vi "Control main.vi"(11 "chosen  distance":dbl) -> ()   [LabVIEW 2015]
uses:
  <vilib>/myRIO/Instrument Drivers/Onboard IO/PWM/typedefs/PWM Reference.ctl
  <vilib>/myRIO/Common/Instrument Driver Framework/Utilities/typedefs/myRIO Generic Hardware Reference.ctl
  <vilib>/myRIO/Common/Instrument Driver Framework/Utilities/typedefs/Hardware Version Enum.ctl
  <vilib>/myRIO/Common/Instrument Driver Framework/Utilities/typedefs/myRIO v1.0 Reference.ctl
  <vilib>/myRIO/Common/Instrument Driver Framework/Utilities/typedefs/Generic FPGA Reference.ctl
  <vilib>/myRIO/Common/Instrument Driver Framework/myRIO v1.0/PWM/typedefs/PWM Channels Enum.ctl
  <vilib>/myRIO/Instrument Drivers/Onboard IO/PWM/typedefs/PWM Configuration.ctl
  <vilib>/userdefined/High Color/nirio_resource_hc.ctl
  <vilib>/myRIO/Common/Instrument Driver Framework/Utilities/vis/Is FPGA Ref Available.vi
  <vilib>/myRIO/Common/Instrument Driver Framework/myRIO v1.0/PWM/vis/myRIO v1.1 Open PWM.vi
  <vilib>/myRIO/Instrument Drivers/Onboard IO/PWM/vis/Set Duty Cycle and Frequency.vi
  <vilib>/myRIO/Common/Instrument Driver Framework/Utilities/vis/Validate Channels.vi
  <vilib>/myRIO/Common/Instrument Driver Framework/myRIO v1.0/PWM/vis/myRIO v1.0 Reserve PWM.vi
  <vilib>/myRIO/Common/Instrument Driver Framework/myRIO v1.0/PWM/vis/myRIO v1.0 Build MUX Configuration PWM.vi
  <vilib>/myRIO/Common/Instrument Driver Framework/myRIO v1.0/Resource Manager/vis/myRIO v1.0 Reserve Channel List.vi
  <vilib>/myRIO/Common/Instrument Driver Framework/myRIO v1.0/Resource Manager/vis/myRIO v1.0 Create Configuration List.vi
  <vilib>/myRIO/Common/Instrument Driver Framework/myRIO v1.0/Resource Manager/vis/myRIO v1.0 Reserve Channel.vi
  <vilib>/myRIO/Common/Instrument Driver Framework/myRIO v1.0/Resource Manager/vis/myRIO v1.0 Unreserve Channel.vi
  <vilib>/myRIO/Common/Instrument Driver Framework/myRIO v1.0/Resource Manager/vis/myRIO v1.0 Build Mutex Name.vi
  <vilib>/Utility/VariantDataType/GetNumericInfo.vi
  <vilib>/Utility/error.llb/Error Cluster From Error Code.vi
  <vilib>/myRIO/Common/Instrument Driver Framework/myRIO v1.0/myRIO v1.1 Open.vi
  <vilib>/myRIO/Common/Instrument Driver Framework/Utilities/vis/IO Manager.vi
  <vilib>/myRIO/Common/Instrument Driver Framework/Utilities/vis/Configuration Manager.vi
  <vilib>/myRIO/Common/Instrument Driver Framework/myRIO v1.0/Resource Manager/vis/myRIO v1.0 Configure IO.vi
  <vilib>/myRIO/Common/Instrument Driver Framework/myRIO v1.0/myRIO v1.0 Close.vi
  <vilib>/myRIO/Common/Instrument Driver Framework/myRIO v1.0/PWM/vis/myRIO v1.0 Write PWM.vi
  <vilib>/myRIO/Express VI/Onboard IO/PWM/PWM Express VI.xnode
  <vilib>/myRIO/Instrument Drivers/Onboard IO/PWM/vis/myRIO PWM Open.xnode
  <vilib>/myRIO/Instrument Drivers/Onboard IO/PWM/PWM.lvlib
panel:
  in  "error in (no error) 2":errorcluster
  out "error out 5":errorcluster
  out "error out 4":errorcluster
  out "Current location":dbl
  out "First location":dbl
  out "Final location":dbl
  out "remainder":dbl
  out "error out":errorcluster
  in  "error in (no error)":errorcluster
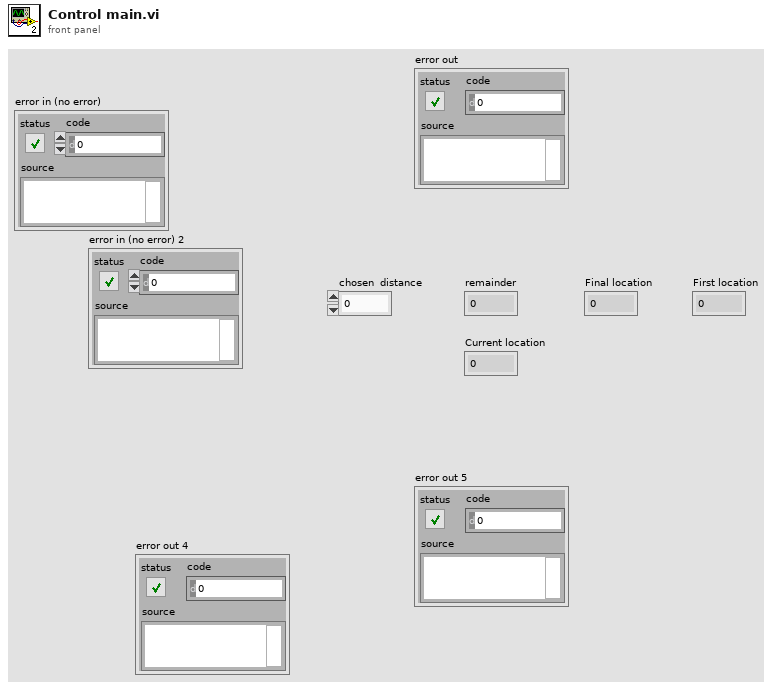
[diagram p1: front panel]
types:
  T1 = typedef "PWM.lvlib/PWM Reference.ctl" = cluster{"myRIO Reference":T2, "PWM Channels Enum":T6, "PWM Configuration":T7}
  T2 = typedef "myRIO Generic Hardware Reference.ctl" = cluster{"myRIO Model":T3, "myRIO Hardware Reference":T4}
  T3 = typedef "Hardware Version Enum.ctl" = enum16{"Unknown", "myRIO-1900", "myRIO-1950", "roboRIO"}
  T4 = typedef "myRIO v1.0 Reference.ctl" = cluster{"Generic FPGA Reference":T5, "Allow multiple opens":bool}
  T5 = typedef "Generic FPGA Reference.ctl" = refnum<k20>
  T6 = typedef "PWM Channels Enum.ctl" = enum16{"Not Connected", "C/PWM0", "C/PWM1", "A/PWM0", "A/PWM1", "A/PWM2", "B/PWM0", "B/PWM1", "B/PWM2", "PWM/PWM0", "PWM/PWM1", "PWM/PWM2", "PWM/PWM3", "PWM/PWM4", "PWM/PWM5", "PWM/PWM6", "PWM/PWM7", "PWM/PWM8", "PWM/PWM9"}
  T7 = typedef "PWM.lvlib/PWM Configuration.ctl" = cluster{"Frequency":dbl, "Duty Cycle":dbl}
  T8 = typedef "nirio_resource_hc.ctl" = tag
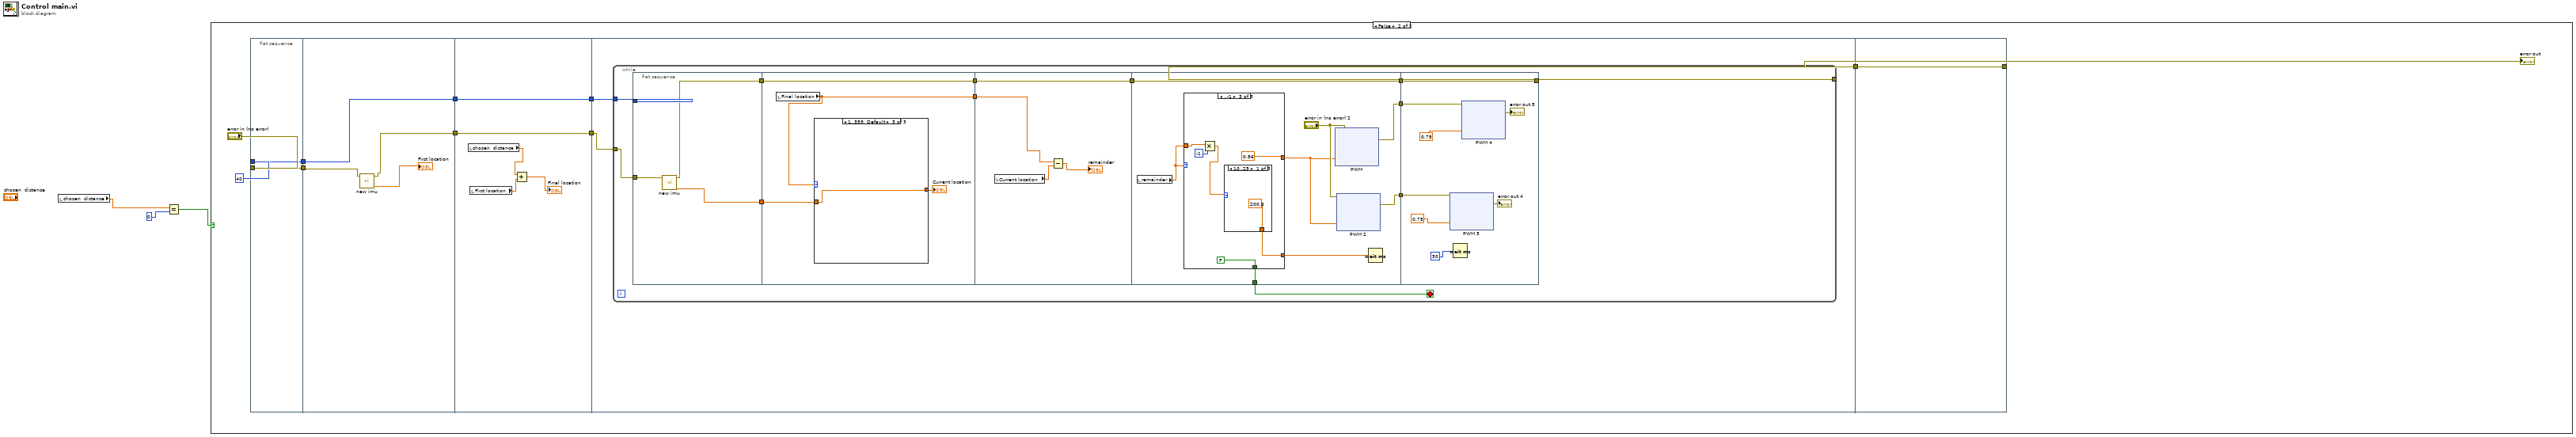
[diagram p0: block diagram]
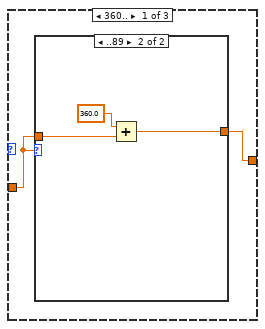
[diagram p3: hidden frame]
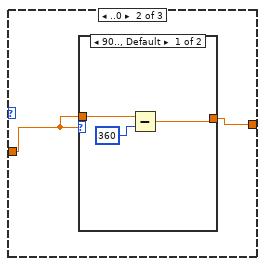
[diagram p5: hidden frame]
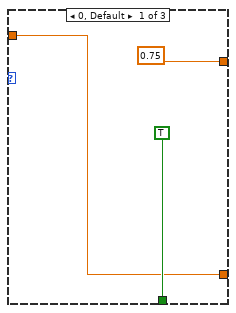
[diagram p7: hidden frame]
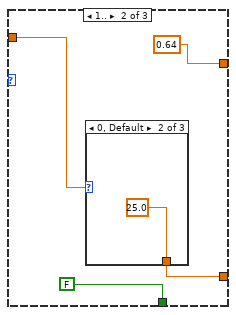
[diagram p8: hidden frame]
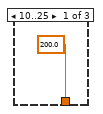
[diagram p9: hidden frame]
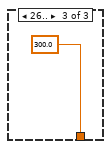
[diagram p10: hidden frame]
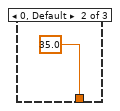
[diagram p11: hidden frame]
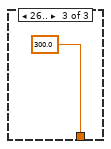
[diagram p12: hidden frame]
diagram:
  n1 = local read "chosen  distance"() -> (w1:dbl)
  n2 = Equal?(x=w1, y=0) -> (x = y?=w3:bool)
  n3 = case shown="False" w3 {
    frame True {
    }
    frame False {
      n4 = flat-sequence {
        tunnel: u8 40 ("Slave Address (7-bit)") -> [w14]
        tunnel: "error in (no error)" -> [w15]
        tunnel: [w15] -> w5
        tunnel: [w14] -> w4
        tunnel: [w17] -> w13
        tunnel: [w19] -> w12
        tunnel: w5 -> [w18]
        tunnel: w4 -> [w19]
        tunnel: w13 -> [w24]
        tunnel: [w24] -> w11
        tunnel: w12 -> [w21]
        tunnel: [w21] -> w10
        tunnel: w11 -> [w27]
        tunnel: w10 -> [w26]
        tunnel: [w25] -> w9
        tunnel: [w239] -> w6
        tunnel: w9 -> [w239]
        frame #0 {
        }
        frame #1 {
          n5 = call "new imu.vi"("error in (no error)"=w18) -> ("Numeric"=→"First location":dbl, "error out"=w17:errorcluster)  [unwired: 9 in]
        }
        frame #2 {
          n6 = local read "chosen  distance"() -> (w20:dbl)
          n7 = local read "First location"() -> (w23:dbl)
          n8 = Add(x=w20, y=w23) -> (x+y=→"Final location":dbl)
        }
        frame #3 {
          n9 = while {
            tunnel: w27 -> [w31]
            tunnel: [w39] -> w25
            tunnel: w26 -> [w38]
            stop <- w37 stop-if-true
            n10 = flat-sequence {
              tunnel: [w42] -> w35
              tunnel: [w41] -> w32
              tunnel: w38 -> [_]
              tunnel: w31 -> [w40]
              tunnel: w35 -> [w46]
              tunnel: [w46] -> w34
              tunnel: [w45] -> w33
              tunnel: w32 -> [w44]
              tunnel: w34 -> [w63]
              tunnel: [w63] -> w30
              tunnel: w33 -> [w60]
              tunnel: w30 -> [w71]
              tunnel: [w70] -> w37
              tunnel: [w71] -> w36
              tunnel: [w68] -> w29
              tunnel: [w67] -> w28
              tunnel: w36 -> [w168]
              tunnel: [w168] -> w39
              tunnel: w29 -> [w162]
              tunnel: w28 -> [w161]
              frame #0 {
                n11 = call "new imu.vi"("error in (no error)"=w40) -> ("Numeric"=w41:dbl, "error out"=w42:errorcluster)  [unwired: 9 in]
              }
              frame #1 {
                n12 = local read "Final location"() -> (w45:dbl)
                n13 = case shown="1..359, Default" w45 {
                  tunnel: w44 -> [w47 w54 w59]
                  tunnel: [w48 w53 w59] -> w43
                  frame 360.. {
                    n14 = case shown="..89" w47 {
                      tunnel: [w49 w51] -> w48
                      tunnel: w47 -> [w49 w50]
                      frame 90.., Default {
                      }
                      frame ..89 {
                        n15 = Add(x=360.0, y=w50) -> (x+y=w51:dbl)
                      }
                    }
                  }
                  frame ..0 {
                    n16 = case shown="90.., Default" w54 {
                      tunnel: [w57 w58] -> w53
                      tunnel: w54 -> [w56 w58]
                      frame 90.., Default {
                        n17 = Subtract(x=w56, y=360) -> (x-y=w57:dbl)
                      }
                      frame ..89 {
                      }
                    }
                  }
                  frame 1..359, Default {
                  }
                }
                "Current location" <- w43
              }
              frame #2 {
                n18 = local read "Current location"() -> (w62:dbl)
                n19 = Subtract(x=w60, y=w62) -> (x-y=→"remainder":dbl)
              }
              frame #3 {
                n20 = local read "remainder"() -> (w65:dbl)
                n21 = case shown="..-1" w65 {
                  tunnel: [TRUE FALSE FALSE] -> w70
                  tunnel: [0.75 0.64 0.86] -> w66
                  tunnel: w65 -> [w142 w145 w155]
                  tunnel: [w142 w146 w153] -> w64
                  frame 0, Default {
                  }
                  frame 1.. {
                    n22 = case shown="0, Default" w145 {
                      tunnel: [200.0 25.0 300.0] -> w146
                      frame 10..25 {
                      }
                      frame 0, Default {
                      }
                      frame 26.. {
                      }
                    }
                  }
                  frame ..-1 {
                    n23 = Multiply(x=w155, y=-1) -> (x*y=w152:dbl)
                    n24 = case shown="10..25" w152 {
                      tunnel: [200.0 35.0 300.0] -> w153
                      frame 10..25 {
                      }
                      frame 0, Default {
                      }
                      frame 26.. {
                      }
                    }
                  }
                }
                n25 = xnode "PWM"("Duty Cycle"=w66, "error in (no error)"="error in (no error) 2") -> ("error out"=w68:errorcluster)
                n26 = xnode "PWM 2"("Duty Cycle"=w66, "error in (no error)"="error in (no error) 2") -> ("error out"=w67:errorcluster)
                n27 = Wait (ms)(milliseconds to wait=w64) -> ()  [unwired: 1 out]
              }
              frame #4 {
                n28 = xnode "PWM 3"("Duty Cycle"=0.75, "error in (no error)"=w161) -> ("error out"=→"error out 4":errorcluster)
                n29 = Wait (ms)(milliseconds to wait=50) -> ()  [unwired: 1 out]
                n30 = xnode "PWM 4"("Duty Cycle"=0.75, "error in (no error)"=w162) -> ("error out"=→"error out 5":errorcluster)
              }
            }
          }
        }
        frame #4 {
        }
      }
      "error out" <- w6
    }
  }
